vi "Dashboard Main.vi"() -> ()   [LabVIEW 2020]
uses:
  Auto Selector.ctl
  <vilib>/Utility/miscctls.llb/LVRowAndColumnTypeDef.ctl
  <vilib>/event_ctls.llb/eventvkey.ctl
  <vilib>/Rock Robotics/Network Tables/NT Read Numeric Array.vi
  <vilib>/Rock Robotics/Network Tables/NT Read Boolean.vi
  <vilib>/Rock Robotics/WPI/Dashboard/WPI_DashboardLogging Global.vi
panel:
  in  "Camera Settings Right":T1={"Frame Rate"=30, "Compression"=30, "Size"=1, "DB Camera Config"=FALSE} {"Frame Rate" scale=1.0..30.0; "Compression" scale=100.0..-1.0; "Size" items=["640x480", "320x240", "160x120"]}
  in  "Camera Name Right":string(combo)="No Camera Selection"
  in  "Camera Settings":T1={"Frame Rate"=30, "Compression"=30, "Size"=1, "DB Camera Config"=FALSE} {"Frame Rate" scale=1.0..30.0; "Compression" scale=100.0..-1.0; "Size" items=["640x480", "320x240", "160x120"]}
  in  "TCP":refnum<k5>
  in  "Rec Mode":enum32{"Stop", "Record", "Playback"}(radio)
  out "Robot IP":string
  out "Image Message":string="Timeout in Camera Communications"
  in  "Dashboard Tab":T2(tab)
  out "Blind Shot":bool
  out "Blind Intake":bool
  in  "Combo Box":string(combo)="Select Autonomous ..."
  in  "WS RPM":dbl=3500.0
  in  "OC RPM":dbl=900.0
  in  "LP RPM":dbl=3900.0
  out "Control Buttons Connected?":bool
  in  "Select Auto":T3="Select Autonomous ..."
  out "NT Connection":bool
  out "MotorChart R":cluster{"Numeric":dbl, "Numeric":dbl}(graph)
  out "MotorChart L":cluster{"Numeric":dbl, "Numeric":dbl}(graph)
  out "MotorSliders R":cluster{"MotorSlide1":dbl, "MotorSlide2":dbl} {"MotorSlide2" scale=-1.0..1.0 scale format="%#_2e"; "MotorSlide1" scale=-1.0..1.0 scale format="%#_2e"}
  out "MotorSliders L":cluster{"MotorSlide1":dbl, "MotorSlide2":dbl} {"MotorSlide2" scale=-1.0..1.0 scale format="%#_2e"; "MotorSlide1" scale=-1.0..1.0 scale format="%#_2e"}
  out "JS1 Z":dbl(slide) scale=-1.0..1.0 scale format="%#_2e"
  out "JS1 Graph":cluster{"X":dbl, "Y":dbl}[](graph)
  out "JS1 Buttons":T4
  out "JS2 Z":dbl(slide) scale=-1.0..1.0 scale format="%#_2e"
  out "JS2 Graph":cluster{"X":dbl, "Y":dbl}[](graph)
  out "JS2 Buttons":T4
  out "Mode":T5(ring)=enum."Auto Disabled"
  out "Right Camera Perf":cluster{"Bandwidth (Mbps)":dbl, "FPS":dbl}
  out "Camera Perf":string
  out "RPM":dbl
  out "BB1":bool
  out "BB 2":bool
  out "ML":bool
  in  "RPM Control":dbl=3400.0
  out "Invert":bool
  out "Slowmode":bool
  in  "Encoder Dist":dbl=80000.0
  out "Missed Mag":bool
  out "RPM Good":bool
  in  "Limelight On":bool
  out "Camera Image Right":T6(plugin-control)
  in  "DB/String 9":string
  in  "DB/String 8":string
  in  "DB/String 7":string
  in  "DB/String 6":string
  in  "DB/String 5":string
  in  "DB/String 4":string
  in  "DB/String 3":string
  in  "DB/String 2":string
  in  "DB/String 1":string
  in  "DB/String 0":string
  in  "DB/Slider 0":dbl(slide) scale=0.0..5.0
  in  "DB/Slider 1":dbl(slide) scale=0.0..5.0
  in  "DB/Slider 2":dbl(slide) scale=0.0..5.0
  in  "DB/Slider 3":dbl(slide) scale=0.0..5.0
  out "DB/LED 3":bool
  out "DB/LED 2":bool
  out "DB/LED 1":bool
  out "DB/LED 0":bool
  in  "DB/Button 3":bool
  in  "DB/Button 2":bool
  in  "DB/Button 1":bool
  in  "DB/Button 0":bool caption="New Name"
  in  "Test Slider":dbl(slide) scale=0.0..100.0 scale format="%#_3g"
  in  "On/Off":bool caption="Solenoid"
  in  "Test Name":u16(ring) items=["Select the test to run..."]
  in  "Test Tree":string(tree)
  in  "Motor":cluster{"Value":dbl, "Enable":bool} {"Value" scale=-1.0..1.0 scale format="%#_3g"}
  out "Progress":T7 {"Test Progress" scale=0.0..100.0}
  in  "Rev/Fwd":cluster{"Forward":bool, "Reverse":bool}
  in  "Test Ring":u16(ring) items=["Monochrome", "Color"]
  out "Cmd Status":string
  in  "Execute Command":bool
  in  "Command Params":string[][](table)
  in  "Command Selection":i32(listbox)
  in  "CheckList":i32(listbox)
  out "Tree":string(tree)
  out "Camera Image":T6(plugin-control)
  out "Background":bool
  in  "Camera Name":string(combo)="No Camera Selection"
  # "HW"
  # "HW"
  # "Joysticks"
  # "Drive Motors"
  # "Front"
  # "Right"
  # "Left"
  # "Back"
  # "This tab is a great place for autonomous settings and robot-specific values.\nPlace controls and indicators inside this tab and match name to\nDashboard Variables on robot. You can also delete this comment."
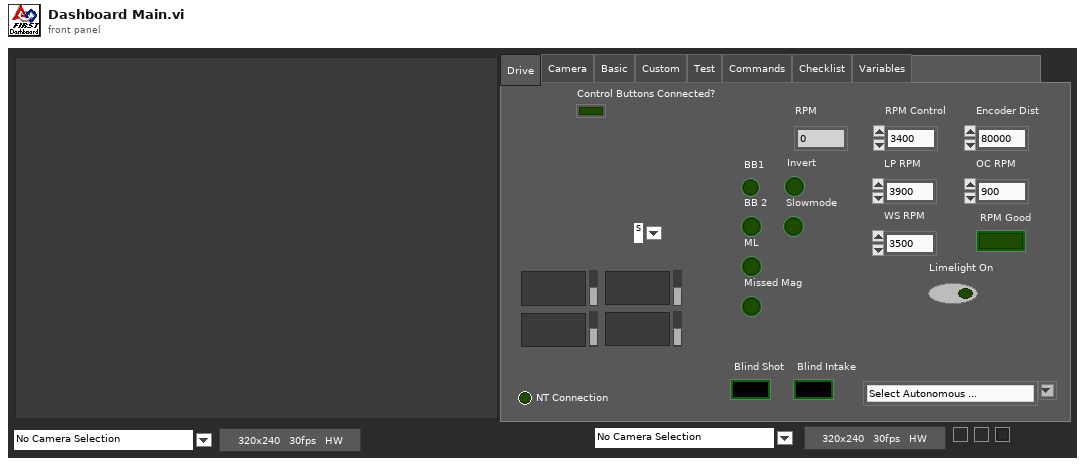
[diagram p1: front panel]
types:
  T1 = cluster{"Frame Rate":i32, "Compression":i32, "Size":u16, "DB Camera Config":bool}
  T2 = enum32{"Drive", "Camera", "Basic", "Custom", "Test", "Commands", "Checklist", "Variables"}
  T3 = typedef "Auto Selector.ctl" = string
  T4 = cluster{bool, bool, bool, bool, bool, bool, bool, bool, bool, bool, bool, bool}
  T5 = enum8{"Tele-Op Disabled", "Tele-Op Enabled", "Auto Disabled", "Auto Enabled", "Test Disabled", "Test Enabled", "Disconnected", "No Code", "E-Stop"}
  T6 = typedef "IMAQ Image.ctl" = refnum<image>
  T7 = cluster{"Test Progress":u8, "Test Progress Text":string}
  T8 = cluster{"Save Path":path, "Interval (s)":dbl, "Keep":i32}
  T9 = typedef "Image Type" = u32
  T10 = cluster{"IDs":cluster{"RPC field ID":u16, "Unique ID":u16}, "String":string}
  T11 = cluster{"Global Rectangle":i32[], "Contours":cluster{"Contour Type":u32, "ROI Type":u32, "Points":i32[]}[]}
  T12 = cluster{"Camera Name":string, string, "Saved DB Images Info":cluster{"Save Path":path, "Interval (s)":dbl, "Keep":i32}}
  T13 = cluster{"Camera Image":refnum<vi>, "Dashboard Tab":refnum<vi>, "Background":refnum<vi>, "Rec Mode":refnum<vi>, "Test Slider":refnum<vi>, "On/Off ":refnum<vi>, "Test Ring":refnum<vi>, "Rev/Fwd":refnum<vi>, "Test Name":refnum<vi>, "Motor":refnum<vi>, "Progress":refnum<vi>, "CheckList":refnum<vi>, "Tree":refnum<vi>, "Test Tree":refnum<vi>, "Command Params":refnum<vi>, "Command Selection":refnum<vi>, "Execute Command":refnum<vi>, "Cmd Status":refnum<vi>, "Camera Settings":refnum<vi>, "Camera Name":refnum<vi>, "Camera Perf":refnum<vi>, "Camera Settings Right":refnum<vi>, "Camera Name Right":refnum<vi>, "Camera Image Right":refnum<vi>}
  T14 = cluster{"Error Strings":string, "Disable Counts":cluster{u16, u16}, "Rail Faults":cluster{u16, u16, u16}, "Robot IP":string, "DB Mode":u8, "Event Info":cluster{"Name":string, "Type":u8, "Number":u16, "Replay":u8}}
  T15 = cluster{"Storage":cluster{"Disk Free":u64, "RAM Block":u32, "RAM free":u32}, "CPU Utilization":cluster{"CPU % ISR":sgl, "CPU % Time Crit":sgl, "CPU % Timed Str":sgl, "CPU % High":sgl, "CPU % Above":sgl, "CPU % Normal":sgl, "CPU % Low":sgl}, "CAN":cluster{"% Bus Utilization":sgl, "Bus Off Cnt":u32, "TX_FIFO Full Cnt":u32, "Receive Error Cnt":u8, "Transmit Error Cnt":u8}, "HID":cluster{"HID Outputs":u32, "Rumble Low":u16, "Rumble High":u16}[]}
  T16 = cluster{"Status bits":cluster{"Test Mode":bool, "Autonomous":bool, "Enabled":bool, "Code Start":bool, "Brownout":bool, "Reserved 2":bool, "Reserved 3":bool, "E-Stop":bool}, "Code Trace":cluster{"Disabled":bool, "TeleOp":bool, "Auto":bool, "Test":bool}, "Controller Type":enum16{"unknown", "cRIO", "roboRio"}, "Code?":enum16{"unknown", "noCode", "code"}, "Battery V":dbl}
  T17 = cluster{"Control Bits":cluster{"TestMode":bool, "Autonomous":bool, "Enabled":bool, "FMS Present":bool, bool, bool, bool, "E-Stop":bool}, "Team Station ":u8, "Countdown":sgl, "Joystick Values":cluster{"Axes":dbl[], "Buttons":bool[], "POVs":i16[]}[]}
  T18 = cluster{"Axes":dbl[], "Buttons":bool[], "POVs":i16[]}[]
  T19 = cluster{"Axes":dbl[], "Buttons":bool[], "POVs":i16[]}
  T20 = cluster{"Buttons[0]":bool, "Buttons[1]":bool, "Buttons[2]":bool, "Buttons[3]":bool, "Buttons[4]":bool, "Buttons[5]":bool, "Buttons[6]":bool, "Buttons[7]":bool, "Buttons[8]":bool, "Buttons[9]":bool, "Buttons[10]":bool, "Buttons[11]":bool}
  T21 = cluster{"Camera Name Right":string, string, "Saved DB Images Info":cluster{"Save Path":path, "Interval (s)":dbl, "Keep":i32}}
  T22 = cluster{"Operation":enum16{"Update", "Clear"}, "Color Box":u32}[]
  T23 = typedef "eventvkey.ctl" = enum16{"ASCII", "Enter", "Return", "Shift", "Ctrl", "Alt", "Cmd", "Opt", "Caps", "NumLock", "Clear", "Break", "Up", "Down", "Left", "Right", "Insert", "Delete", "Home", "End", "PageUp", "PageDown", "Escape", "Help", "Pause", "ScrollLock", "F1", "F2", "F3", "F4", "F5", "F6", "F7", "F8", "F9", "F10", "F11", "F12", "F13", "F14", "F15", "F16", "F17", "F18", "F19", "F20", "F21", "F22", "F23", "F24", "Play", "VolumeUp", "VolumeDown", "Mute", "Two Byte Char"}
  T24 = cluster{"Image Size":bool, "Image Type":bool, "Pixel Value":bool, "ROI Information":bool, "Zoom Factor":bool}
  T25 = cluster{"Operation":enum16{"Update", "Clear"}, "Color Box":u32}
  T26 = typedef "LVRowAndColumnTypeDef.ctl" = cluster{"Row":i32, "Column":i32}
  T27 = cluster{"Shift":bool, "Ctrl":bool, "Alt":bool, "Cmd":bool, "Opt":bool}
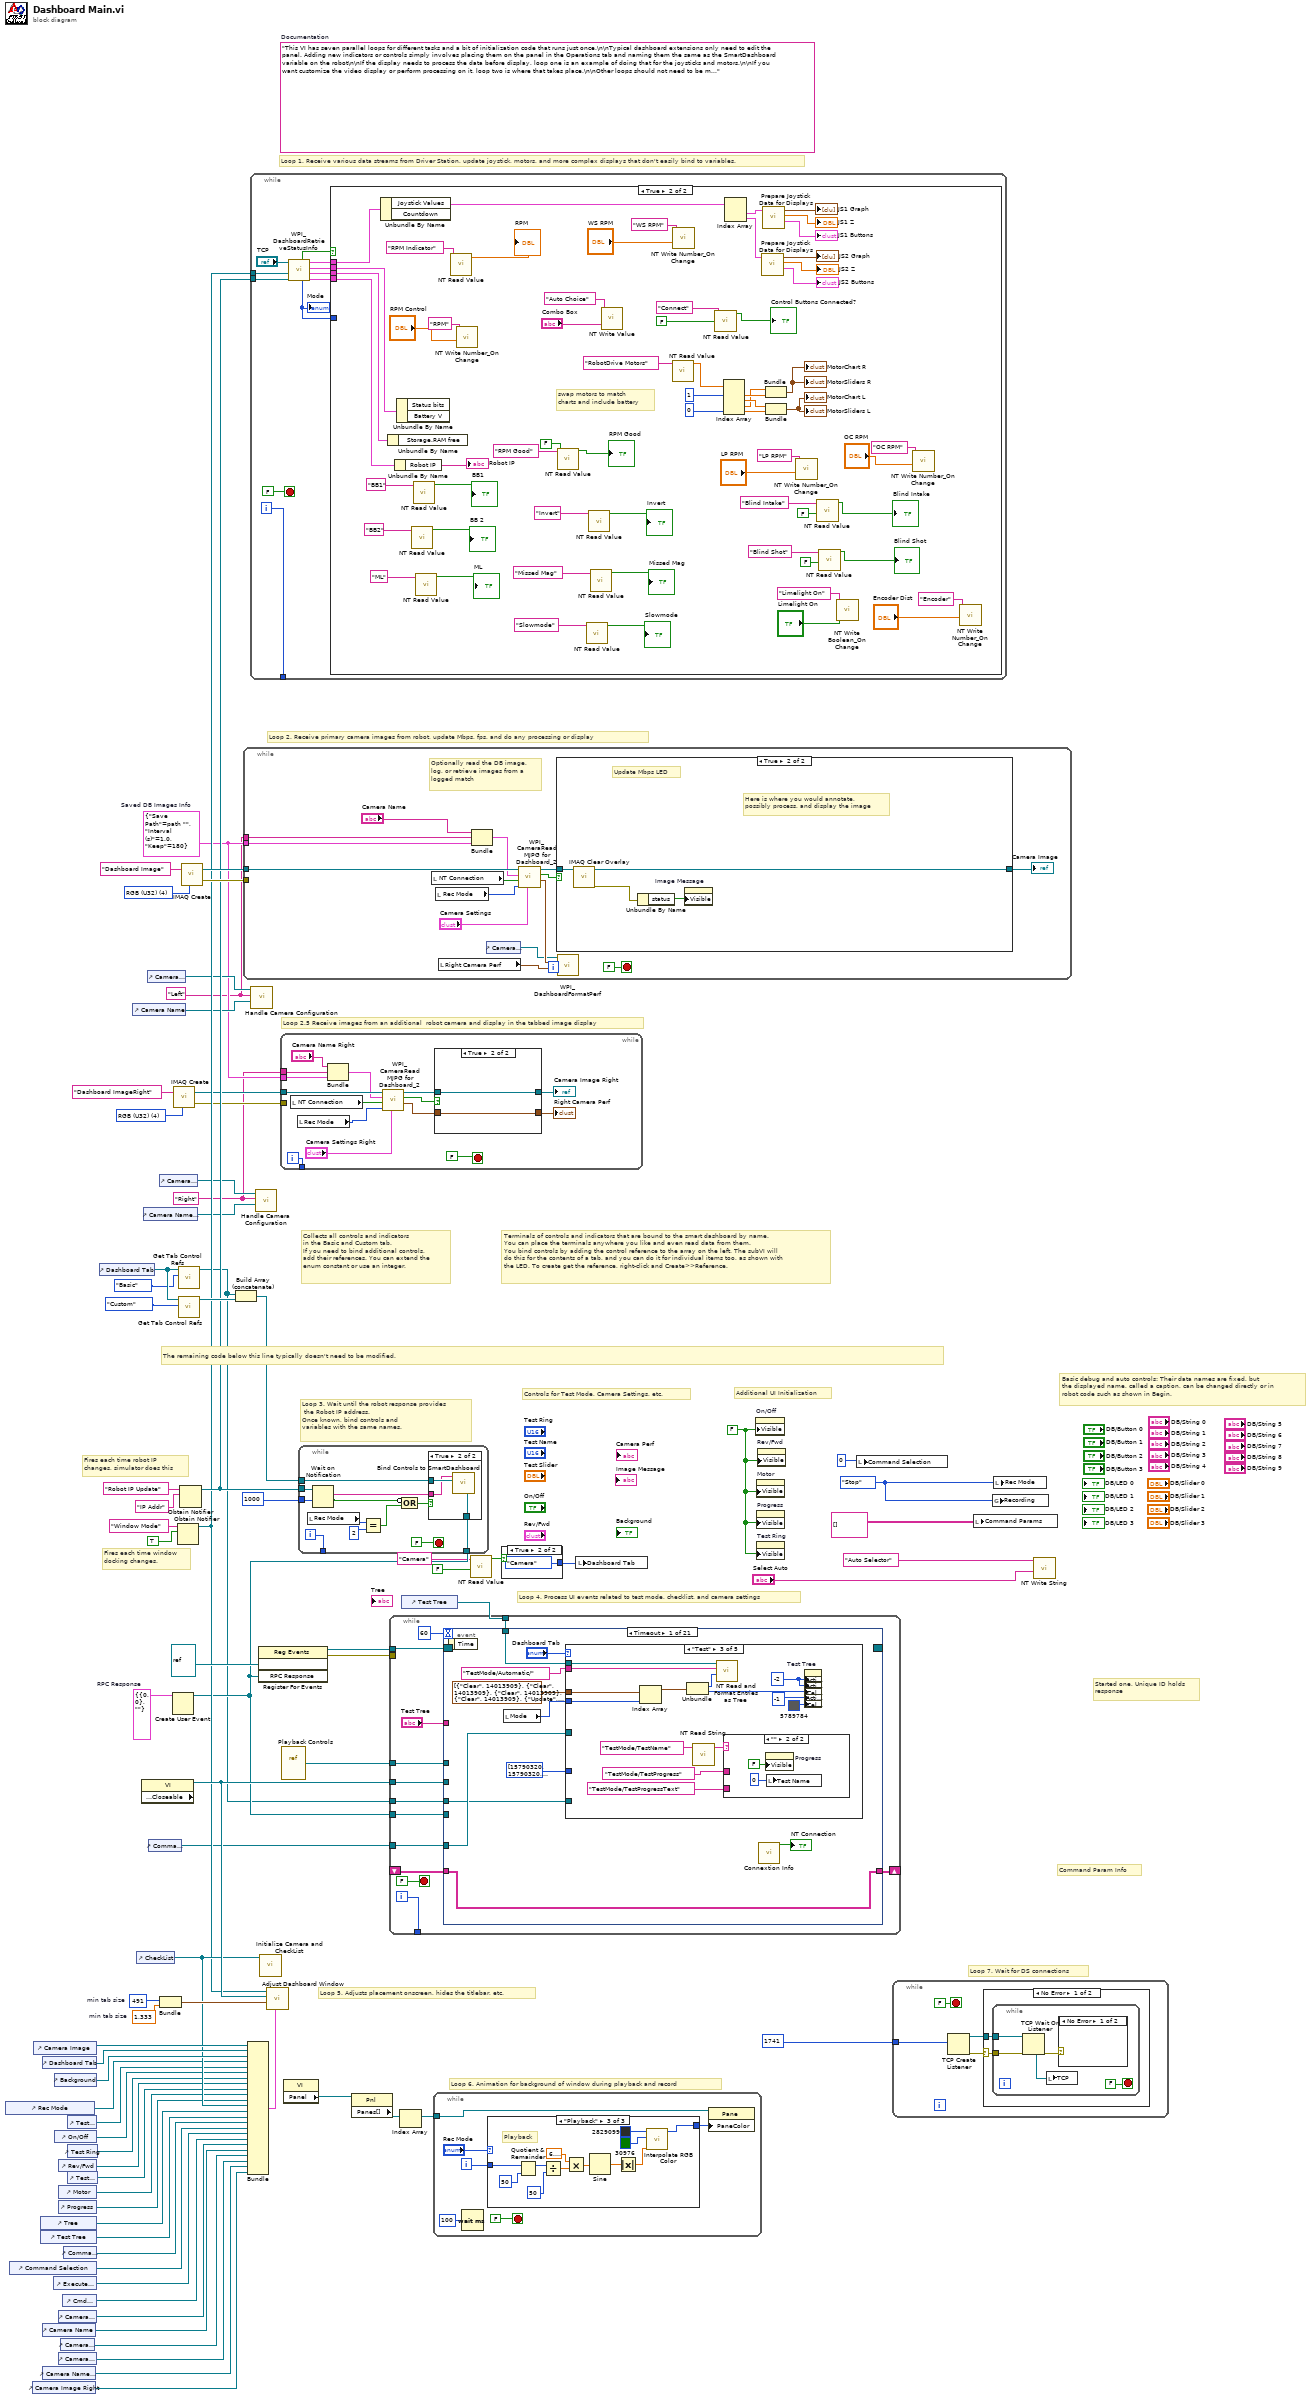
[diagram p0: block diagram]
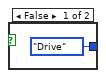
[diagram p2: hidden frame]
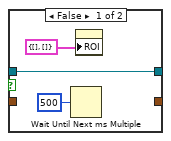
[diagram p3: hidden frame]
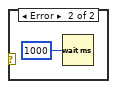
[diagram p4: hidden frame]
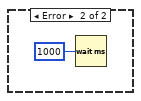
[diagram p5: hidden frame]
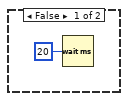
[diagram p6: hidden frame]
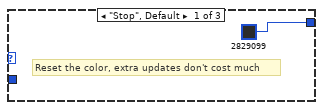
[diagram p7: hidden frame]
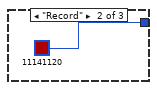
[diagram p8: hidden frame]
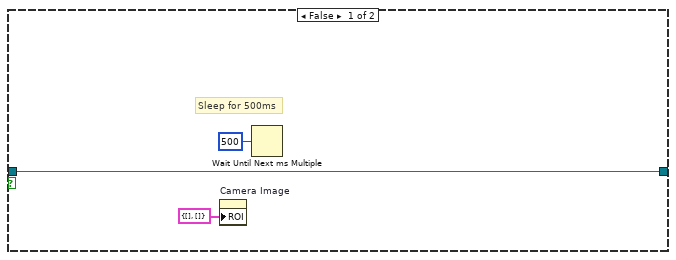
[diagram p10: hidden frame]
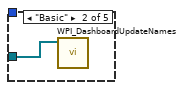
[diagram p12: hidden frame]
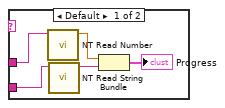
[diagram p13: hidden frame]
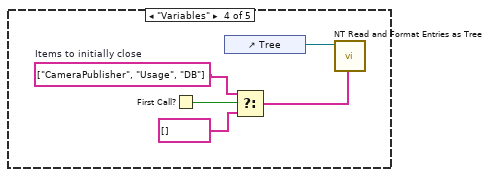
[diagram p14: hidden frame]
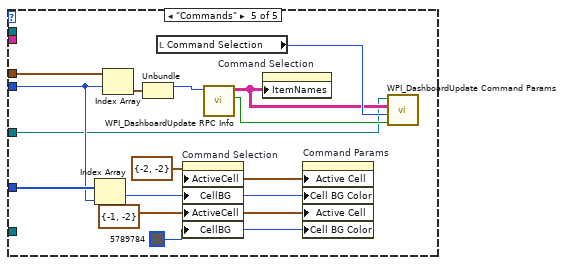
[diagram p15: hidden frame]
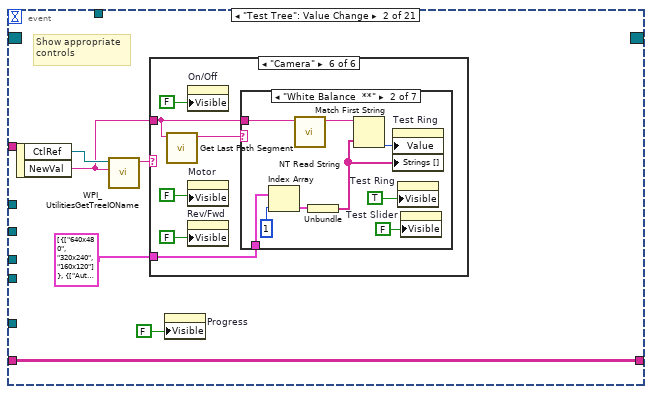
[diagram p16: hidden frame]
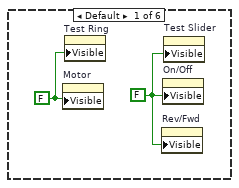
[diagram p17: hidden frame]
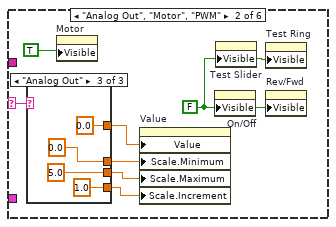
[diagram p18: hidden frame]
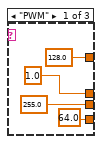
[diagram p19: hidden frame]
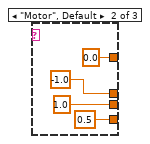
[diagram p20: hidden frame]
diagram:
  w7 = T8 {"Save Path"=path "", "Interval (s)"=1.0, "Keep"=180}  # Saved DB Images Info
  w6 = "Right"
  w5 = "Left"
  w17 = T9 4 items=["Grayscale (U8)", "Grayscale (I16)", "Grayscale (SGL)", "Complex (CSG)", "RGB (U32)", "HSL (U32)", "RGB (U64)"] ("Image Type")
  w32 = T10 {"IDs"={"RPC field ID"=0, "Unique ID"=0}, "String"=""}  # RPC Response
  w55 = 491  # min tab size
  w54 = 1.333  # min tab size
  w62 = enum32{"Stop", "Record", "Playback"}."Stop" ("Rec Mode")
  w39 = FALSE ("Visible")
  (unwired) "This VI has seven parallel loops for different tasks and a bit of initialization code that runs just once.\n\nTypical dashboard extensions only need to edit the panel. Adding new indicators or controls simply involves placing them on the panel in the Operations tab and naming them the same as the SmartDashboard variable on the robot\n\nIf the display needs to process the data before display, loop one is an example of doing that for the joysticks and motors.\n\nIf you want customize the video display or perform processing on it, loop two is where that takes place.\n\nOther loops should not need to be modified. They are pretty standard, and document the task they perform."  # Documentation
  w79 = T9 4 items=["Grayscale (U8)", "Grayscale (I16)", "Grayscale (SGL)", "Complex (CSG)", "RGB (U32)", "HSL (U32)", "RGB (U64)"] ("Image Type")
  # "Loop 2.5 Receive images from an additional  robot camera and display in the tabbed image display"
  # "Command Param Info"
  # "Started one, Unique ID holds\nresponse"
  # "Loop 7. Wait for DS connections"
  # "Basic debug and auto controls: Their data names are fixed, but\nthe displayed name, called a caption, can be changed directly or in\nrobot code such as shown in Begin."
  # "Controls for Test Mode, Camera Settings, etc."
  # "Additional UI Initialization"
  # "Loop 6. Animation for background of window during playback and record"
  # "Fires each time robot IP\nchanges, simulator does this"
  # "Fires each time window\ndocking changes."
  # "Collects all controls and indicators\nin the Basic and Custom tab.\nIf you need to bind additional controls,\nadd their references. You can extend the\nenum constant or use an integer."
  # "The remaining code below this line typically doesn't need to be modified."
  # "Loop 4. Process UI events related to test mode, checklist, and camera settings"
  # "Terminals of controls and indicators that are bound to the smart dashboard by name.\nYou can place the terminals anywhere you like and even read data from them.\nYou bind controls by adding the control reference to the array on the left. The subVI will\ndo this for the contents of a tab, and you can do it for individual items too, as shown with\nthe LED. To create get the reference, right-click and Create>>Reference."
  # "Loop 3. Wait until the robot response provides\n the Robot IP address.\nOnce known, bind controls and\nvariables with the same names."
  # "Loop 5. Adjusts placement onscreen, hides the titlebar, etc."
  # "Loop 1. Receive various data streams from Driver Station, update joystick, motors, and more complex displays that don't easily bind to variables."
  # "Loop 2. Receive primary camera images from robot, update Mbps, fps, and do any processing or display"
  n1 = control-ref of="Rec Mode"() -> (w45:refnum<vi>)
  n2 = control-ref of="Command Selection"() -> (w31:refnum<vi>)
  n3 = control-ref of="Camera Image Right"() -> (w10:refnum<vi>)
  n4 = control-ref of="Camera Image"() -> (w57:refnum<vi>)
  n5 = control-ref of="Tree"() -> (w49:refnum<vi>)
  n6 = control-ref of="Test Tree"() -> (w48:refnum<vi>)
  n7 = control-ref of="Dashboard Tab"() -> (w56:refnum<vi>)
  n8 = control-ref of="Camera Name"() -> (w4:refnum<vi>)
  n9 = control-ref of="Camera Name Right"() -> (w11:refnum<vi>)
  n10 = control-ref of="Execute Command"() -> (w33:refnum<vi>)
  n11 = control-ref of="Background"() -> (w52:refnum<vi>)
  n12 = control-ref of="On/Off"() -> (w43:refnum<vi>)
  n13 = control-ref of="Progress"() -> (w40:refnum<vi>)
  n14 = control-ref of="Camera Settings"() -> (w23:refnum<vi>)
  n15 = control-ref of="Camera Settings Right"() -> (w12:refnum<vi>)
  n16 = control-ref of="Rev/Fwd"() -> (w41:refnum<vi>)
  n17 = control-ref of="Motor"() -> (w46:refnum<vi>)
  n18 = control-ref of="Camera Perf"() -> (w22:refnum<vi>)
  n19 = control-ref of="Cmd Status"() -> (w27:refnum<vi>)
  n20 = control-ref of="Command Params"() -> (w34:refnum<vi>)
  n21 = control-ref of="Test Slider"() -> (w44:refnum<vi>)
  n22 = control-ref of="Test Ring"() -> (w42:refnum<vi>)
  n23 = control-ref of="Test Name"() -> (w47:refnum<vi>)
  n24 = control-ref of="Dashboard Tab"() -> (w60:refnum<vi>)
  n25 = control-ref of="Camera Name"() -> (w24:refnum<vi>)
  n26 = control-ref of="CheckList"() -> (w50:refnum<vi>)
  n27 = property class="VI" props=["Front Panel.Closeable"]() -> (reference out=w61:refnum<vi>)  [unwired: 2 in, 2 out]
  n28 = control-ref of="Camera Name Right"() -> (w13:refnum<vi>)
  n29 = control-ref of="Camera Settings"() -> (w25:refnum<vi>)
  n30 = control-ref of="Command Params"() -> (w26:refnum<vi>)
  n31 = control-ref of="Camera Settings Right"() -> (w14:refnum<vi>)
  n32 = Bundle("min tab size"=w55, "min tab size"=w54) -> (w53:cluster{"min tab size":i32, "min tab size":dbl})  [unwired: 1 in]
  n33 = Create User Event(user event datatype=w32) -> (user event=w28:refnum<user-event>)  [unwired: 1 in, 1 out]
  n34 = call "IMAQ Create"("Image Name"="Dashboard ImageRight", "Image Type"=w17) -> ("New Image"=w16:T6, "error out"=w15:errorcluster)  [unwired: 2 in, 1 out]
  n35 = Obtain Notifier(name (unnamed)="Window Mode", notification data type=TRUE) -> (notifier out=w37:refnum<notifier>)  [unwired: 2 in, 2 out]
  n36 = call <vilib>:"Get Tab Control Refs.vi"("Page Index"=T2."Basic" ("Dashboard Tab"), "TabControl in"=w60) -> ("ControlsOnPage"=w21:refnum<vi>[])  [unwired: 9 in]
  n37 = call <vilib>:"Get Tab Control Refs.vi"("Page Index"=T2."Custom" ("Dashboard Tab"), "TabControl in"=w60) -> ("ControlsOnPage"=w59:refnum<vi>[])  [unwired: 9 in]
  n38 = Obtain Notifier(name (unnamed)="Robot IP Update", notification data type="IP Addr" ("name (unnamed)")) -> (notifier out=w38:refnum<notifier>)  [unwired: 2 in, 2 out]
  n39 = call "IMAQ Create"("Image Name"="Dashboard Image", "Image Type"=w79) -> ("New Image"=w77:T6, "error out"=w76:errorcluster)  [unwired: 2 in, 1 out]
  n40 = Build Array (concatenate)(w21, w59) -> (w58:refnum<vi>[])
  n41 = while {
    tunnel: w77 -> [w93]
    tunnel: w76 -> [_]
    tunnel: w7 -> [w86]
    tunnel: w5 -> [w84]
    stop <- FALSE stop-if-true
    # "Optionally read the DB image,\nlog, or retrieve images from a\nlogged match"
    n42 = local read "NT Connection"() -> (w87:bool)
    n43 = local read "Rec Mode"() -> (w90:enum32{"Stop", "Record", "Playback"})
    n44 = local read "Right Camera Perf"() -> (w82:cluster{"Bandwidth (Mbps)":dbl, "FPS":dbl})
    n45 = Bundle("Camera Name"="Camera Name", w84, "Saved DB Images Info"=w86) -> (w85:T12)  [unwired: 1 in]
    n46 = control-ref of="Camera Perf"() -> (w81:refnum<vi>)
    n47 = call <vilib>:"WPI_CameraRead MJPG for Dashboard_2.vi"("Camera Settings"="Camera Settings", "Rec Mode"=w90, "NT Connection"=w87, "Capture Info"=w85, "Image in"=w93) -> ("perf info"=w83:cluster{"Bandwidth (Mbps)":dbl, "fps":dbl}, "Active"=w91:bool, "Image\\ out"=w92:T6)  [unwired: 4 in]
    n48 = case shown="True" w91 {
      tunnel: w92 -> [w96 w99]
      tunnel: [w96 w98] -> w88
      frame False {
        # "Sleep for 500ms"
        n49 = property on="Camera Image" class="ImageControl"("ROI"=T11 {"Global Rectangle"=[], "Contours"=[]}) -> ()  [unwired: 2 in, 2 out]
        n50 = Wait Until Next ms Multiple(millisecond multiple=u32 500) -> ()  [unwired: 1 out]
      }
      frame True {
        # "Here is where you would annotate,\npossibly process, and display the image"
        # "Update Mbps LED"
        n51 = call "IMAQ Clear Overlay"("Image"=w99) -> ("error out"=w100:errorcluster, "Image Out"=w98:T6)  [unwired: 2 in, 7 out]
        n52 = Unbundle By Name(w100) -> ("status"=w101:bool)
        n53 = property on="Image Message" class="Str"("Visible"=w101) -> ()  [unwired: 2 in, 2 out]
      }
    }
    "Camera Image" <- w88
    n54 = call <vilib>:"WPI_DashboardFormatPerf.vi"("Right Camera Perf"=w82, "Performance"=w83, "String in"=w81) -> ()  [unwired: 9 in]
  }
  n55 = Bundle("Camera Image"=w57, "Dashboard Tab"=w56, "Background"=w52, "Rec Mode"=w45, "Test Slider"=w44, "On/Off"=w43, "Test Ring"=w42, "Rev/Fwd"=w41, "Test Name"=w47, "Motor"=w46, "Progress"=w40, "CheckList"=w50, "Tree"=w49, "Test Tree"=w48, "Command Params"=w34, "Command Selection"=w31, "Execute Command"=w33, "Cmd Status"=w27, "Camera Settings"=w23, "Camera Name"=w4, "Camera Perf"=w22, "Camera Settings Right"=w12, "Camera Name Right"=w11, "Camera Image Right"=w10) -> (w51:T13)  [unwired: 1 in]
  n56 = while {
    tunnel: [w111] -> _
    tunnel: w38 -> [w105]
    tunnel: w37 -> [w102]
    i -> [w111]
    stop <- FALSE stop-if-true
    n57 = call <vilib>:"WPI_DashboardRetrieveStatusInfo.vi"("Binding Refnum"=w105, "Window Mode Notifier"=w102, "TCP Cnx"="TCP") -> ("Power and Errors"=w106:T14, "Robot Metrics"=w109:T15, "Status Info"=w110:T16, "Control Info"=w107:T17, "Robot Mode"=w104:T5, "Process?"=w108:bool)  [unwired: 3 in]
    "Mode" <- w104
    n58 = case shown="True" w108 {
      tunnel: w110 -> [_ w177]
      tunnel: w109 -> [_ w176]
      tunnel: w107 -> [_ w175]
      tunnel: w106 -> [_ w174]
      tunnel: w104 -> [_ _]
      frame False {
        n59 = Wait (ms)(milliseconds to wait=u32 20) -> ()  [unwired: 1 out]
      }
      frame True {
        # "swap motors to match\ncharts and include battery"
        n60 = Unbundle By Name(w175) -> ("Joystick Values"=w165:T18)  [unwired: 1 out]
        n61 = Unbundle By Name(w176) -> ()  [unwired: 1 out]
        n62 = Unbundle By Name(w174) -> ("Robot IP"=→"Robot IP":string)
        n63 = Unbundle By Name(w177) -> ()  [unwired: 2 out]
        n64 = call-poly <vilib>:"NT Read Value.vi"("Name"="BB2") -> ("Boolean"=→"BB 2":bool)  [unwired: 9 in, 1 out]
        n65 = call-poly <vilib>:"NT Read Value.vi"("Name"="BB1") -> ("Boolean"=→"BB1":bool)  [unwired: 9 in, 1 out]
        n66 = call-poly <vilib>:"NT Read Value.vi"("Name"="ML") -> ("Boolean"=→"ML":bool)  [unwired: 9 in, 1 out]
        n67 = call-poly <vilib>:"NT Read Value.vi"("Name"="RPM Indicator") -> ("Numeric"=→"RPM":dbl)  [unwired: 9 in, 1 out]
        n68 = call "NT Write Number_On Change.vi"("Numeric"="RPM Control", "Name"="RPM") -> ()  [unwired: 9 in, 1 out]
        n69 = call-poly <vilib>:"NT Read Value.vi"("Default Value"=FALSE, "Name"="RPM Good") -> ("Boolean"=→"RPM Good":bool)  [unwired: 8 in, 1 out]
        n70 = call-poly <vilib>:"NT Read Value.vi"("Name"="Slowmode") -> ("Boolean"=→"Slowmode":bool)  [unwired: 9 in, 1 out]
        n71 = call-poly <vilib>:"NT Read Value.vi"("Name"="Invert") -> ("Boolean"=→"Invert":bool)  [unwired: 9 in, 1 out]
        n72 = call-poly <vilib>:"NT Read Value.vi"("Name"="Missed Mag") -> ("Boolean"=→"Missed Mag":bool)  [unwired: 9 in, 1 out]
        n73 = call-poly <vilib>:"NT Write Value.vi"("String"="Combo Box", "Name"="Auto Choice") -> ()  [unwired: 9 in, 1 out]
        n74 = call-poly <vilib>:"NT Read Value.vi"("Name"="RobotDrive Motors") -> ("Numeric Array"=w155:dbl[])  [unwired: 9 in, 1 out]
        n75 = call "NT Write Number_On Change.vi"("Numeric"="WS RPM", "Name"="WS RPM") -> ()  [unwired: 9 in, 1 out]
        n76 = call-poly <vilib>:"NT Read Value.vi"("Default Value"=FALSE, "Name"="Connect") -> ("Boolean"=→"Control Buttons Connected?":bool)  [unwired: 8 in, 1 out]
        n77 = Index Array(array=w155, index #1=1, index #4=0) -> (element #1=w169:dbl, element #2=w170:dbl, element #3=w168:dbl, element #4=w173:dbl)  [unwired: 2 in]
        n78 = Index Array(array=w165) -> (element #1=w164:T19, element #2=w160:T19)  [unwired: 2 in]
        n79 = call "Prepare Joystick Data for Displays.vi"("Joystick Values"=w160) -> ("Buttons"=→"JS2 Buttons":T20, "Z Axis"=→"JS2 Z":dbl, "Cartesian Data"=→"JS2 Graph":cluster{"X axis":dbl, "X axis":dbl}[])  [unwired: 8 in]
        n80 = call "Prepare Joystick Data for Displays.vi"("Joystick Values"=w164) -> ("Buttons"=→"JS1 Buttons":T20, "Z Axis"=→"JS1 Z":dbl, "Cartesian Data"=→"JS1 Graph":cluster{"X axis":dbl, "X axis":dbl}[])  [unwired: 8 in]
        n81 = Bundle("Numeric"=w168, "Numeric"=w169) -> (→"MotorChart R" →"MotorSliders R":cluster{"Numeric":dbl, "Numeric":dbl})  [unwired: 1 in]
        n82 = Bundle("Numeric"=w170, "Numeric"=w173) -> (→"MotorChart L" →"MotorSliders L":cluster{"Numeric":dbl, "Numeric":dbl})  [unwired: 1 in]
        n83 = call "NT Write Number_On Change.vi"("Numeric"="LP RPM", "Name"="LP RPM") -> ()  [unwired: 9 in, 1 out]
        n84 = call-poly <vilib>:"NT Read Value.vi"("Default Value"=FALSE, "Name"="Blind Intake") -> ("Boolean"=→"Blind Intake":bool)  [unwired: 8 in, 1 out]
        n85 = call-poly <vilib>:"NT Read Value.vi"("Default Value"=FALSE, "Name"="Blind Shot") -> ("Boolean"=→"Blind Shot":bool)  [unwired: 8 in, 1 out]
        n86 = call "NT Write Boolean_On Change.vi"("Boolean"="Limelight On", "Name"="Limelight On") -> ()  [unwired: 9 in, 1 out]
        n87 = call "NT Write Number_On Change.vi"("Numeric"="OC RPM", "Name"="OC RPM") -> ()  [unwired: 9 in, 1 out]
        n88 = call "NT Write Number_On Change.vi"("Numeric"="Encoder Dist", "Name"="Encoder") -> ()  [unwired: 9 in, 1 out]
      }
    }
  }
  n89 = call "Handle Camera Configuration.vi"("CameraNameRef"=w24, "Display Name"=w5, "ClusterRef"=w25) -> ()  [unwired: 9 in]
  n90 = call "Handle Camera Configuration.vi"("CameraNameRef"=w13, "Display Name"=w6, "ClusterRef"=w14) -> ()  [unwired: 9 in]
  n91 = register-events(refnum<vi> refnum, w28) -> (reference out=w66:refnum<event-registration>, error out=w65:errorcluster)  [unwired: 2 in]
  n92 = call "Initialize Camera and CheckList.vi"("ListBox in"=w50) -> ()  [unwired: 11 in]
  n93 = call "Adjust Dashboard Window.vi"("Sizing Refnums"=w51, "Size Constraints"=w53, "VI"=w61, "WIn Mode"=w37) -> ()  [unwired: 8 in]
  n94 = while {
    tunnel: w16 -> [w192]
    tunnel: w15 -> [_]
    tunnel: [w187] -> _
    tunnel: w7 -> [w183]
    tunnel: w6 -> [w180]
    i -> [w187]
    stop <- FALSE stop-if-true
    n95 = local read "NT Connection"() -> (w184:bool)
    n96 = local read "Rec Mode"() -> (w191:enum32{"Stop", "Record", "Playback"})
    n97 = Bundle("Camera Name Right"="Camera Name Right", w180, "Saved DB Images Info"=w183) -> (w182:T21)  [unwired: 1 in]
    n98 = call <vilib>:"WPI_CameraRead MJPG for Dashboard_2.vi"("Camera Settings"="Camera Settings Right", "Rec Mode"=w191, "NT Connection"=w184, "Capture Info"=w182, "Image in"=w192) -> ("perf info"=w178:cluster{"Bandwidth (Mbps)":dbl, "fps":dbl}, "Active"=w186:bool, "Image\\ out"=w189:T6)  [unwired: 4 in]
    n99 = case shown="True" w186 {
      tunnel: w189 -> [w194 w197]
      tunnel: [w194 w197] -> w185
      tunnel: [_ w196] -> w179
      tunnel: w178 -> [_ w196]
      frame False {
        n100 = Wait Until Next ms Multiple(millisecond multiple=u32 500) -> ()  [unwired: 1 out]
        n101 = property on="Camera Image Right" class="ImageControl"("ROI"=T11 {"Global Rectangle"=[], "Contours"=[]}) -> ()  [unwired: 2 in, 2 out]
      }
      frame True {
      }
    }
    "Camera Image Right" <- w185
    "Right Camera Perf" <- w179
  }
  n102 = vi-ref "Playback Controls.vi"() -> (w67:refnum<vi>)
  n103 = property class="VI"() -> ("Panel"=w69:refnum<vi>)  [unwired: 2 in, 2 out]
  n104 = while {
    tunnel: w58 -> [w209]
    tunnel: w38 -> [w207]
    tunnel: [w205] -> _
    tunnel: u32 1000 ("milliseconds to wait") -> [w204]
    tunnel: w28 -> [w198]
    i -> [w205]
    stop <- FALSE stop-if-true
    n105 = local read "Rec Mode"() -> (w200:enum32{"Stop", "Record", "Playback"})
    n106 = Wait on Notification(notifier=w207, timeout in ms (-1)=w204) -> (notification=w206:string, timed out?=w202:bool)  [unwired: 2 in, 2 out]
    n107 = Equal?(x=w200, y=u16 2 ("Rec Mode")) -> (x = y?=w201:bool)
    n108 = Compound Arithmetic op=OR(invert w202, w201) -> (w203:bool)
    n109 = case shown="True" w203 {
      tunnel: w209 -> [_ w212]
      tunnel: w206 -> [_ w211]
      tunnel: w198 -> [_ w210]
      frame False {
      }
      frame True {
        n110 = call <vilib>:"Bind Controls to SmartDashboard.vi"("RPC ref"=w210, "Bound Control Refs"=w212, "Server IP Address"=w211) -> ()  [unwired: 9 in]
      }
    }
  }
  n111 = property class="Pnl"(reference=w69) -> ("Panes[]"=w70:refnum<vi>[])  [unwired: 1 in, 2 out]
  n112 = Index Array(array=w70) -> (element=w68:refnum<vi>)  [unwired: 1 in]
  n113 = control-ref of="Test Tree"() -> (w71:refnum<vi>)
  n114 = while {
    tunnel: [w222] -> _
    tunnel: w71 -> [w221]
    tunnel: w67 -> [w220]
    tunnel: w66 -> [w219]
    tunnel: w65 -> [_]
    tunnel: w61 -> [w218]
    tunnel: w28 -> [w217]
    tunnel: w26 -> [w216]
    shift-right: [w215] -> _
    shift-left: _ -> [w214]
    tunnel: w21 -> [w213]
    i -> [w222]
    stop <- FALSE stop-if-true
    n115 = event shown="[0] Timeout" {
      selector: w219 -> [_ _ _ _ _ _ _ _ _ _ _ _ _ _ _ _ _ _ _ _ _]
      dyn-events: [_ _ _ _ _ _ _ _ _ _ _ _ _ _ _ _ w482 _ _ _ _] -> _
      timeout: u32 60 ("milliseconds to wait") -> [_ _ _ _ _ _ _ _ _ _ _ _ _ _ _ _ _ _ _ _ _]
      tunnel: w221 -> [w234 _ _ _ _ _ _ _ _ _ _ _ _ _ _ _ _ _ _ _ _]
      tunnel: "Test Tree" -> [_ _ _ _ _ _ _ _ _ _ _ w449 w457 w459 w463 w471 _ _ _ _ _]
      tunnel: w220 -> [_ _ _ _ _ _ _ _ _ _ _ _ _ _ _ _ w484 _ w502 _ _]
      tunnel: w218 -> [_ _ _ _ _ _ _ _ _ _ _ _ _ _ _ _ w480 _ _ _ _]
      tunnel: w217 -> [_ _ _ _ _ _ _ _ _ _ _ _ _ _ _ _ w478 _ _ _ _]
      tunnel: w216 -> [w229 _ _ _ _ _ w400 _ _ _ _ _ _ _ _ _ _ _ _ _ _]
      tunnel: [w228 w277 w379 w384 w393 w397 w398 w407 w417 w424 w436 w448 w455 w458 w462 w470 w477 w497 w499 w503 w516] -> w215
      tunnel: w214 -> [w228 w277 w379 w384 w393 w397 w398 _ _ w424 w436 w448 w455 w458 w462 w470 w477 w497 w499 w503 w516]
      tunnel: w213 -> [w226 _ _ _ _ _ _ _ _ _ _ _ _ _ _ _ _ _ _ _ _]
      event Timeout {
        n116 = event-data() -> ()  [unwired: 1 in, 1 out]
        n117 = local read "Mode"() -> (w231:T5)
        n118 = case shown="\"Test\"" "Dashboard Tab" {
          tunnel: w234 -> [_ _ w250 _ _]
          tunnel: "TestMode/Automatic/" ("Name Pattern") -> [_ _ w249 _ _]
          tunnel: T22 [{"Operation"=enum."Clear", "Color Box"=14013909}, {"Operation"=enum."Clear", "Color Box"=14013909}, {"Operation"=enum."Clear", "Color Box"=14013909}, {"Operation"=enum."Clear", "Color Box"=14013909}, {"Operation"=enum."Update", "Color Box"=14013909}, {"Operation"=enum."Update", "Color Box"=16777215}, {"Operation"=enum."Clear", "Color Box"=14013909}, {"Operation"=enum."Clear", "Color Box"=14013909}, {"Operation"=enum."Clear", "Color Box"=14013909}] -> [_ _ w242 _ w270]
          tunnel: w231 -> [_ _ w241 _ w269]
          tunnel: u32[] [15790320, 15790320, 15790320, 15790320, 16777215, 16777215, 15790320, 15790320, 15790320] -> [_ _ _ _ w275]
          tunnel: w229 -> [_ _ _ _ w263]
          tunnel: w226 -> [_ w236 _ _ _]
          frame "Custom", Default {
          }
          frame "Basic" {
            n119 = call <vilib>:"WPI_DashboardUpdateNames.vi"("Controls on Tab"=w236) -> ()  [unwired: 11 in]
          }
          frame "Test" {
            w248 = -2 ("Active Item:Row Number")
            n120 = Index Array(array=w242, index=w241) -> (element=w243:T25)
            n121 = Unbundle(w243) -> ("Operation"=w244:enum16{"Update", "Clear"}, "Color Box"=w245:u32)
            n122 = call <vilib>:"NT Read String.vi"("Name"="TestMode/TestName") -> ("String"=w239:string)  [unwired: 9 in, 1 out]
            n123 = call <vilib>:"NT Read and Format Entries as Tree.vi"("Operation"=w244, "Name Pattern"=w249, "Tree Refnum"=w250) -> ()  [unwired: 7 in, 2 out]
            n124 = case shown="\"\"" w239 {
              tunnel: "TestMode/TestProgress" ("Name") -> [w252 _]
              tunnel: "TestMode/TestProgressText" ("Name") -> [w251 _]
              frame Default {
                n125 = call <vilib>:"NT Read Number.vi"("Name"=w252) -> ("Numeric"=w253:dbl)  [unwired: 9 in, 1 out]
                n126 = call <vilib>:"NT Read String.vi"("Name"=w251) -> ("String"=w254:string)  [unwired: 9 in, 1 out]
                n127 = Bundle("Numeric"=w253, "String"=w254) -> (→"Progress":cluster{"Numeric":dbl, "String":string})  [unwired: 1 in]
              }
              frame "" {
                n128 = property on="Progress" class="Clust (strict)"("Visible"=FALSE) -> ()  [unwired: 2 in, 2 out]
                n129 = local write "Test Name"(u16 0) -> ()
              }
            }
            n130 = property on="Test Tree" class="Tree (strict)"("Active Item Row Number"=w248, "ActiveColNum"=w248, "CellBG"=w245, "Active Item Row Number"=-1 ("Active Item:Row Number"), "CellBG"=u32 5789784 ("Color Box")) -> ()  [unwired: 2 in, 2 out]
          }
          frame "Variables" {
            w260 = string[] ["CameraPublisher", "Usage", "DB"]  # Items to initially close
            n131 = First Call?() -> (First Call?: T/F=w261:bool)
            n132 = control-ref of="Tree"() -> (w262:refnum<vi>)
            n133 = Select(t=w260, s=w261, f=string[] []) -> (s? t:f=w258:string[])
            n134 = call <vilib>:"NT Read and Format Entries as Tree.vi"("Tags to  Close"=w258, "Tree Refnum"=w262) -> ()  [unwired: 8 in, 2 out]
          }
          frame "Commands" {
            w271 = u32 5789784 ("Color Box")
            w272 = T26 {"Row"=-1, "Column"=-2} ("Active Cell:Active Cell")
            w274 = T26 {"Row"=-2, "Column"=-2} ("Active Cell:Active Cell")
            n135 = Index Array(array=w275, index=w269) -> (element=w273:u32)
            n136 = Index Array(array=w270, index=w269) -> (element=w268:T25)
            n137 = Unbundle(w268) -> ("Operation"=w267:enum16{"Update", "Clear"})  [unwired: 1 out]
            n138 = local read "Command Selection"() -> (w266:i32)
            n139 = property on="Command Selection" class="MCListbox (strict)"("ActiveCell"=w274, "CellBG"=w273, "ActiveCell"=w272, "CellBG"=w271) -> ()  [unwired: 2 in, 2 out]
            n140 = call <vilib>:"WPI_DashboardUpdate RPC Info.vi"("Operation"=w267) -> ("update"=w265:bool, "commands"=w264:string[][])  [unwired: 9 in]
            n141 = property on="Command Selection" class="MCListbox (strict)"("ItemNames"=w264) -> ()  [unwired: 2 in, 2 out]
            n142 = property on="Command Params" class="Tbl (strict)"("Active Cell"=w274, "Cell BG Color"=w273, "Active Cell"=w272, "Cell BG Color"=w271) -> ()  [unwired: 2 in, 2 out]
            n143 = call <vilib>:"WPI_DashboardUpdate Command Params.vi"("Update"=w265, "NewVal"=w266, "Commands"=w264, "Param Tbl"=w263) -> ()  [unwired: 7 in, 1 out]
          }
        }
        n144 = call <vilib>:"Connextion Info.vi"() -> ("Connected"=→"NT Connection":bool)  [unwired: 10 in, 1 out]
      }
      event "Test Tree": Value Change {
        # "Show appropriate\ncontrols"
        n145 = event-data() -> ("CtlRef"=w280:refnum<vi>, "NewVal"=w278:string)  [unwired: 1 in]
        n146 = call <vilib>:"WPI_UtilitiesGetTreeIOName.vi"("NewVal"=w278, "TreeControl in"=w280) -> ("I/O Name"=w281:string)  [unwired: 9 in]
        n147 = case shown="\"Camera\"" w281 {
          selector: w281 -> [_ w288 _ w310 w319 _]
          tunnel: w278 -> [_ _ w307 w309 _ w326]
          tunnel: cluster{string[]}[] [{["640x480", "320x240", "160x120"]}, {["Auto", "Fixed indoor", "Fixed outdoor 1", "Fixed outdoor 2", "Fixed fluorescent 1", "Fixed fluorescent 2", "Hold current"]}, {["Auto", "Flicker-free 50 Hz", "Flicker-free 60 Hz", "Hold current"]}, {["None", "Prioritize frame rate", "Prioritize image quality"]}, {["Monochrome", "Color"]}] -> [_ _ _ _ _ w325]
          frame Default {
            w283 = FALSE ("Visible")
            w282 = FALSE ("Visible")
            n148 = property on="Motor" class="Clust (strict)"("Visible"=w282) -> ()  [unwired: 2 in, 2 out]
            n149 = property on="Test Ring" class="Ring (strict)"("Visible"=w282) -> ()  [unwired: 2 in, 2 out]
            n150 = property on="Rev/Fwd" class="Clust (strict)"("Visible"=w283) -> ()  [unwired: 2 in, 2 out]
            n151 = property on="On/Off" class="Bool (strict)"("Visible"=w283) -> ()  [unwired: 2 in, 2 out]
            n152 = property on="Test Slider" class="Slide (strict)"("Visible"=w283) -> ()  [unwired: 2 in, 2 out]
          }
          frame "Analog Out", "Motor", "PWM" {
            w289 = FALSE ("Visible")
            n153 = case shown="\"Analog Out\"" w288 {
              tunnel: [1.0 ("Value") -1.0 ("Value") 0.0 ("Value")] -> w287
              tunnel: [255.0 ("Value") 1.0 ("Value") 5.0 ("Value")] -> w286
              tunnel: [128.0 ("Value") 0.0 ("Value") 0.0 ("Value")] -> w285
              tunnel: [64.0 ("Value") 0.5 ("Value") 1.0 ("Value")] -> w284
              frame "PWM" {
              }
              frame "Motor", Default {
              }
              frame "Analog Out" {
              }
            }
            n154 = property on="Motor" class="Clust (strict)"("Visible"=TRUE) -> ()  [unwired: 2 in, 2 out]
            n155 = property on="Value" class="Slide (strict)"("Value"=w285, "Scale.Minimum"=w287, "Scale.Maximum"=w286, "Scale.Increment"=w284) -> ()  [unwired: 2 in, 2 out]
            n156 = property on="On/Off" class="Bool (strict)"("Visible"=w289) -> ()  [unwired: 2 in, 2 out]
            n157 = property on="Test Slider" class="Slide (strict)"("Visible"=w289) -> ()  [unwired: 2 in, 2 out]
            n158 = property on="Test Ring" class="Ring (strict)"("Visible"=w289) -> ()  [unwired: 2 in, 2 out]
            n159 = property on="Rev/Fwd" class="Clust (strict)"("Visible"=w289) -> ()  [unwired: 2 in, 2 out]
          }
          frame "Servo" {
            w305 = FALSE ("Visible")
            n160 = call <vilib>:"NT Read Number.vi"("Name"=w307) -> ("Numeric"=w306:dbl)  [unwired: 9 in, 1 out]
            n161 = property on="Test Slider" class="Slide (strict)"("Visible"=TRUE, "Scale.Maximum"=170.0 ("Scale.Range:Maximum")) -> ()  [unwired: 2 in, 2 out]
            n162 = local write "Test Slider"(w306) -> ()
            n163 = property on="Motor" class="Clust (strict)"("Visible"=w305) -> ()  [unwired: 2 in, 2 out]
            n164 = property on="Rev/Fwd" class="Clust (strict)"("Visible"=w305) -> ()  [unwired: 2 in, 2 out]
            n165 = property on="On/Off" class="Bool (strict)"("Visible"=w305) -> ()  [unwired: 2 in, 2 out]
            n166 = property on="Test Ring" class="Ring (strict)"("Visible"=w305) -> ()  [unwired: 2 in, 2 out]
          }
          frame "Relay", "Solenoid" {
            w308 = FALSE ("Visible")
            n167 = property on="Motor" class="Clust (strict)"("Visible"=w308) -> ()  [unwired: 2 in, 2 out]
            n168 = property on="Test Slider" class="Slide (strict)"("Visible"=w308) -> ()  [unwired: 2 in, 2 out]
            n169 = Search and Replace String(input string=w309, search string="/Value  **", replace string="/Direction") -> (result string=w315:string)  [unwired: 5 in, 3 out]
            n170 = property on="Test Ring" class="Ring (strict)"("Visible"=w308) -> ()  [unwired: 2 in, 2 out]
            n171 = call <vilib>:"NT Read String.vi"("Name"=w315) -> ("String"=w313:string)  [unwired: 9 in, 1 out]
            n172 = Equal?(x="Both directions", y=w313) -> (x = y?=w311:bool)
            n173 = Not(x=w311) -> (.not. x?=w312:bool)
            n174 = property on="Rev/Fwd" class="Clust (strict)"("Visible"=w311) -> ()  [unwired: 2 in, 2 out]
            n175 = property on="On/Off" class="Bool (strict)"("Visible"=w312, "Caption.Text"=w310) -> ()  [unwired: 2 in, 2 out]
          }
          frame "Compressor", "Digital Out" {
            w318 = FALSE ("Visible")
            # "Get direction and finish"
            n176 = property on="Motor" class="Clust (strict)"("Visible"=w318) -> ()  [unwired: 2 in, 2 out]
            n177 = property on="Test Slider" class="Slide (strict)"("Visible"=w318) -> ()  [unwired: 2 in, 2 out]
            n178 = property on="Test Ring" class="Ring (strict)"("Visible"=w318) -> ()  [unwired: 2 in, 2 out]
            n179 = property on="On/Off" class="Bool (strict)"("Visible"=TRUE, "Caption.Text"=w319) -> ()  [unwired: 2 in, 2 out]
            n180 = property on="Rev/Fwd" class="Clust (strict)"("Visible"=FALSE) -> ()  [unwired: 2 in, 2 out]
          }
          frame "Camera" {
            n181 = call <vilib>:"Get Last Path Segment.vi"("String in"=w326) -> ("String out"=w327:string)  [unwired: 10 in]
            n182 = property on="On/Off" class="Bool (strict)"("Visible"=FALSE) -> ()  [unwired: 2 in, 2 out]
            n183 = property on="Motor" class="Clust (strict)"("Visible"=FALSE) -> ()  [unwired: 2 in, 2 out]
            n184 = property on="Rev/Fwd" class="Clust (strict)"("Visible"=FALSE) -> ()  [unwired: 2 in, 2 out]
            n185 = case shown="\"White Balance  **\"" w327 {
              tunnel: w326 -> [w333 w342 w351 w360 w369 _ w375]
              tunnel: w325 -> [w331 w339 w348 w357 w366 _ _]
              frame "Size  **" {
                n186 = Index Array(array=w331) -> (element=w330:cluster{string[]})  [unwired: 1 in]
                n187 = call <vilib>:"NT Read String.vi"("Name"=w333) -> ("String"=w332:string)  [unwired: 9 in, 1 out]
                n188 = Unbundle(w330) -> (w328:string[])
                n189 = Match First String(2:w328, 3:w332) -> (0:w329:i32)  [unwired: 1 out]
                n190 = property on="Test Ring" class="Ring (strict)"("Value"=w329, "Strings []"=w328) -> ()  [unwired: 2 in, 2 out]
                n191 = property on="Test Ring" class="Ring (strict)"("Visible"=TRUE) -> ()  [unwired: 2 in, 2 out]
                n192 = property on="Test Slider" class="Slide (strict)"("Visible"=FALSE) -> ()  [unwired: 2 in, 2 out]
              }
              frame "White Balance  **" {
                n193 = Index Array(array=w339, index=1) -> (element=w340:cluster{string[]})
                n194 = call <vilib>:"NT Read String.vi"("Name"=w342) -> ("String"=w341:string)  [unwired: 9 in, 1 out]
                n195 = Unbundle(w340) -> (w337:string[])
                n196 = Match First String(2:w337, 3:w341) -> (0:w336:i32)  [unwired: 1 out]
                n197 = property on="Test Ring" class="Ring (strict)"("Value"=w336, "Strings []"=w337) -> ()  [unwired: 2 in, 2 out]
                n198 = property on="Test Ring" class="Ring (strict)"("Visible"=TRUE) -> ()  [unwired: 2 in, 2 out]
                n199 = property on="Test Slider" class="Slide (strict)"("Visible"=FALSE) -> ()  [unwired: 2 in, 2 out]
              }
              frame "Exposure  **" {
                n200 = Index Array(array=w348, index=2) -> (element=w349:cluster{string[]})
                n201 = call <vilib>:"NT Read String.vi"("Name"=w351) -> ("String"=w350:string)  [unwired: 9 in, 1 out]
                n202 = Unbundle(w349) -> (w345:string[])
                n203 = Match First String(2:w345, 3:w350) -> (0:w346:i32)  [unwired: 1 out]
                n204 = property on="Test Ring" class="Ring (strict)"("Value"=w346, "Strings []"=w345) -> ()  [unwired: 2 in, 2 out]
                n205 = property on="Test Ring" class="Ring (strict)"("Visible"=TRUE) -> ()  [unwired: 2 in, 2 out]
                n206 = property on="Test Slider" class="Slide (strict)"("Visible"=FALSE) -> ()  [unwired: 2 in, 2 out]
              }
              frame "Exposure Priority  **" {
                n207 = Index Array(array=w357, index=3) -> (element=w358:cluster{string[]})
                n208 = call <vilib>:"NT Read String.vi"("Name"=w360) -> ("String"=w359:string)  [unwired: 9 in, 1 out]
                n209 = Unbundle(w358) -> (w354:string[])
                n210 = Match First String(2:w354, 3:w359) -> (0:w355:i32)  [unwired: 1 out]
                n211 = property on="Test Ring" class="Ring (strict)"("Value"=w355, "Strings []"=w354) -> ()  [unwired: 2 in, 2 out]
                n212 = property on="Test Ring" class="Ring (strict)"("Visible"=TRUE) -> ()  [unwired: 2 in, 2 out]
                n213 = property on="Test Slider" class="Slide (strict)"("Visible"=FALSE) -> ()  [unwired: 2 in, 2 out]
              }
              frame "Color Enable  **" {
                n214 = Index Array(array=w366, index=4) -> (element=w367:cluster{string[]})
                n215 = call <vilib>:"NT Read String.vi"("Name"=w369) -> ("String"=w368:string)  [unwired: 9 in, 1 out]
                n216 = Unbundle(w367) -> (w363:string[])
                n217 = Match First String(2:w363, 3:w368) -> (0:w364:i32)  [unwired: 1 out]
                n218 = property on="Test Ring" class="Ring (strict)"("Value"=w364, "Strings []"=w363) -> ()  [unwired: 2 in, 2 out]
                n219 = property on="Test Ring" class="Ring (strict)"("Visible"=TRUE) -> ()  [unwired: 2 in, 2 out]
                n220 = property on="Test Slider" class="Slide (strict)"("Visible"=FALSE) -> ()  [unwired: 2 in, 2 out]
              }
              frame Default {
                n221 = property on="Test Ring" class="Ring (strict)"("Visible"=FALSE) -> ()  [unwired: 2 in, 2 out]
                n222 = property on="Test Slider" class="Slide (strict)"("Visible"=FALSE) -> ()  [unwired: 2 in, 2 out]
              }
              frame "Brightness  **", "Color Level  **", "Compression  **", "FPS  **", "Sharpness  **" {
                n223 = call <vilib>:"NT Read Number.vi"("Name"=w375) -> ("Numeric"=w374:dbl)  [unwired: 9 in, 1 out]
                n224 = local write "Test Slider"(w374) -> ()
                n225 = property on="Test Slider" class="Slide (strict)"("Visible"=TRUE, "Scale.Maximum"=100.0 ("Scale.Range:Maximum")) -> ()  [unwired: 2 in, 2 out]
                n226 = property on="Test Ring" class="Ring (strict)"("Visible"=FALSE) -> ()  [unwired: 2 in, 2 out]
              }
            }
          }
        }
        n227 = property on="Progress" class="Clust (strict)"("Visible"=FALSE) -> ()  [unwired: 2 in, 2 out]
      }
      event "Test Name": Mouse Enter {
        # "Populate the ring with the list of tests"
        n228 = event-data() -> ()  [unwired: 1 in, 1 out]
        n229 = call <vilib>:"NT Read String Array.vi"("Name"="TestMode/TestList") -> ("String Array"=w383:string[])  [unwired: 9 in, 1 out]
        n230 = Build Array (concatenate)("Select the test to run...", w383) -> (w382:string[])
        n231 = property on="Test Name" class="Ring (strict)"("Strings []"=w382) -> ()  [unwired: 2 in, 2 out]
      }
      event "Test Name": Value Change {
        w385 = FALSE ("Visible")
        # "Tell the robot the test name to run"
        n232 = event-data() -> ("NewVal"=w389:u16)  [unwired: 1 in]
        n233 = property on="Test Name" class="Ring (strict)"() -> ("Strings []"=w390:string[])  [unwired: 2 in, 2 out]
        n234 = local write "Progress"(T7 {"Test Progress"=0, "Test Progress Text"=""} ("Progress")) -> ()
        n235 = Index Array(array=w390, index=w389) -> (element=w388:string)
        n236 = call <vilib>:"NT Write String.vi"("String"=w388, "Name"="TestMode/TestName") -> ()  [unwired: 9 in, 1 out]
        n237 = property on="Progress" class="Clust (strict)"("Visible"=TRUE) -> ()  [unwired: 2 in, 2 out]
        n238 = property on="Motor" class="Clust (strict)"("Visible"=w385) -> ()  [unwired: 2 in, 2 out]
        n239 = property on="Test Slider" class="Slide (strict)"("Visible"=w385) -> ()  [unwired: 2 in, 2 out]
        n240 = property on="On/Off" class="Bool (strict)"("Visible"=w385) -> ()  [unwired: 2 in, 2 out]
        n241 = property on="Rev/Fwd" class="Clust (strict)"("Visible"=w385) -> ()  [unwired: 2 in, 2 out]
        n242 = property on="Test Ring" class="Ring (strict)"("Visible"=w385) -> ()  [unwired: 2 in, 2 out]
      }
      event Mouse Enter {
        # "Populate the combo box with the list of autonomous options"
        n243 = event-data() -> ()  [unwired: 1 in, 1 out]
        n244 = call <vilib>:"NT Read String Array.vi"("Name"="Auto List") -> ("String Array"=w392:string[])  [unwired: 9 in, 1 out]
        n245 = property on="Select Auto" class="CmbBox (strict)"("Strings[]"=w392) -> ()  [unwired: 2 in, 2 out]
      }
      event Value Change {
        # "User modified the Auto Selection. Write to NT variable so robot knows."
        n246 = event-data() -> ("NewVal"=w395:T3)  [unwired: 1 in]
        n247 = call <vilib>:"NT Write String.vi"("String"=w395, "Name"="Auto Selector") -> ()  [unwired: 9 in, 1 out]
      }
      event "Command Selection": Value Change {
        # "Get the params and show in table"
        n248 = event-data() -> ("NewVal"=w401:i32)  [unwired: 1 in]
        n249 = property on="Command Selection" class="MCListbox (strict)"() -> ("ItemNames"=w399:string[][])  [unwired: 2 in, 2 out]
        n250 = call <vilib>:"WPI_DashboardUpdate Command Params.vi"("NewVal"=w401, "Commands"=w399, "Param Tbl"=w400) -> ()  [unwired: 8 in, 1 out]
      }
      event "Execute Command": Value Change {
        # "Started one, Unique ID holds\nresponse"
        n251 = event-data() -> ()  [unwired: 1 in, 1 out]
        n252 = property on="Command Selection" class="MCListbox (strict)"() -> ("ItemNames"=w412:string[][])  [unwired: 2 in, 2 out]
        n253 = Index Array(array=w412, index (row)="Command Selection", index (col)=0) -> (element=w410:string)
        n254 = call <vilib>:"Invoke Commands.vi"("Command Params"="Command Params", "Function Name"=w410) -> ("Params"=w406:u8, "Started"=w405:bool)  [unwired: 7 in, 1 out]
        n255 = Array Subset(array="Command Params", length (row)=w406) -> (w407:string[][])  [unwired: 3 in]
        n256 = Select(t="Executing" ("Cmd Status"), s=w405, f="" ("Cmd Status")) -> (s? t:f=→"Cmd Status":string)
      }
      event "Command Selection": Double Click {
        n257 = event-data() -> ("Row"=w420:i32)  [unwired: 1 in]
        n258 = property on="Command Selection" class="MCListbox (strict)"() -> ("ItemNames"=w423:string[][])  [unwired: 2 in, 2 out]
        n259 = local read "Command Params"() -> (w419:string[][])
        n260 = Index Array(array=w423, index (row)=w420, index (col)=0) -> (element=w421:string)
        n261 = call <vilib>:"Invoke Commands.vi"("Command Params"=w419, "Function Name"=w421) -> ("Params"=w418:u8, "Started"=w413:bool)  [unwired: 7 in, 1 out]
        n262 = Array Subset(array=w419, length (row)=w418) -> (w417:string[][])  [unwired: 3 in]
        n263 = Select(t="Executing" ("Cmd Status"), s=w413, f="" ("Cmd Status")) -> (s? t:f=w414:string)
        n264 = local write "Cmd Status"(w414) -> ()
      }
      event "CheckList": Double Click {
        # "Shift clears all"
        # "Update symbols on the listbox"
        n265 = event-data() -> ("PlatMods.Shift"=w425:bool, "Row"=w427:i32)  [unwired: 1 in]
        n266 = case shown="True" w425 {
          tunnel: w427 -> [w431 _]
          tunnel: 1 -> [w430 _]
          frame False {
            n267 = property on="CheckList" class="LstBox (strict)"() -> ("Item Symbols"=w429:i32[])  [unwired: 2 in, 2 out]
            n268 = Replace Array Subset(array=w429, new element=w430, index=w431) -> (w428:i32[])
            n269 = property on="CheckList" class="LstBox (strict)"("Item Symbols"=w428) -> ()  [unwired: 2 in, 2 out]
          }
          frame True {
            w432 = 0 ("Top Row")
            n270 = property on="CheckList" class="LstBox (strict)"() -> ("Number of Rows"=w434:u32)  [unwired: 2 in, 2 out]
            n271 = Initialize Array(0, w434) -> (w433:i32[])
            n272 = property on="CheckList" class="LstBox (strict)"("Top Row"=w432, "Value"=w432, "Item Symbols"=w433) -> ()  [unwired: 2 in, 2 out]
          }
        }
      }
      event "CheckList": Key Down {
        # "Update symbols on the listbox\nLeft and right keys check and uncheck"
        n273 = event-data() -> ("VKey"=w438:T23)  [unwired: 1 in]
        n274 = case shown="\"Left\", \"Right\"" w438 {
          selector: w438 -> [w443 _]
          tunnel: eventvkey."Left" ("VKey") -> [w441 _]
          frame "Left", "Right" {
            n275 = Equal?(x=w441, y=w443) -> (x = y?=w442:bool)
            n276 = Select(t=0, s=w442, f=1) -> (s? t:f=w444:i32)
            n277 = property on="CheckList" class="LstBox (strict)"() -> ("Item Symbols"=w447:i32[])  [unwired: 2 in, 2 out]
            n278 = Replace Array Subset(array=w447, new element=w444, index="CheckList") -> (w446:i32[])
            n279 = property on="CheckList" class="LstBox (strict)"("Item Symbols"=w446) -> ()  [unwired: 2 in, 2 out]
          }
          frame Default {
          }
        }
      }
      event "Motor.Enable": Value Change {
        # "When the test mode otor enable helper is set, update that\ntree row item's value"
        n280 = event-data() -> ("NewVal"=w453:bool)  [unwired: 1 in]
        n281 = Unbundle("Motor") -> ("Value"=w452:dbl)  [unwired: 1 out]
        n282 = Select(t=w452, s=w453, f=0.0) -> (s? t:f=w450:dbl)
        n283 = call <vilib>:"NT Write Number.vi"("Numeric"=w450, "Name"=w449) -> ()  [unwired: 9 in, 1 out]
      }
      event "Test Slider": Value Change {
        # "When the test mode slider helper is set, update that\ntree row item's value"
        n284 = event-data() -> ("NewVal"=w456:dbl)  [unwired: 1 in]
        n285 = call <vilib>:"NT Write Number.vi"("Numeric"=w456, "Name"=w457) -> ()  [unwired: 9 in, 1 out]
      }
      event "On/Off": Value Change {
        # "When the test mode on/off helper value is set, update that\ntree row item's value"
        n286 = event-data() -> ("NewVal"=w461:bool)  [unwired: 1 in]
        n287 = Boolean To (0,1)(Boolean=w461) -> (0, 1=w460:i16)
        n288 = call <vilib>:"NT Write Number.vi"("Numeric"=w460, "Name"=w459) -> ()  [unwired: 9 in, 1 out]
      }
      event "Rev/Fwd": Value Change {
        # "When the test mode helper value for relays is set, update that\ntree row item's value"
        n289 = event-data() -> ("NewVal.Forward"=w469:bool, "NewVal.Reverse"=w468:bool)  [unwired: 1 in]
        n290 = Boolean To (0,1)(Boolean=w469) -> (0, 1=w465:i16)
        n291 = Boolean To (0,1)(Boolean=w468) -> (0, 1=w467:i16)
        n292 = Negate(x=w467) -> (-x=w466:i16)
        n293 = Add(x=w465, y=w466) -> (x+y=w464:i16)
        n294 = call <vilib>:"NT Write Number.vi"("Numeric"=w464, "Name"=w463) -> ()  [unwired: 9 in, 1 out]
      }
      event "Test Ring": Value Change {
        # "When a test mode helper value is selected from the ring,\nset the tree item's variable to the string value"
        n295 = event-data() -> ("NewVal"=w473:u16)  [unwired: 1 in]
        n296 = property on="Test Ring" class="Ring (strict)"() -> ("Strings []"=w474:string[])  [unwired: 2 in, 2 out]
        n297 = Index Array(array=w474, index=w473) -> (element=w472:string)
        n298 = call <vilib>:"NT Write String.vi"("String"=w472, "Name"=w471) -> ()  [unwired: 9 in, 1 out]
      }
      event "Rec Mode": Value Change {
        # "Update globals for recording mode and path to read log from.\nClear when logging and let NetworkTables set path for vision to\nuse."
        n299 = event-data() -> ("NewVal"=w485:enum32{"Stop", "Record", "Playback"})  [unwired: 1 in]
        n300 = global write "WPI_DashboardLogging Global.vi" "Logging Filename"(path "") -> ()
        n301 = global write "WPI_DashboardLogging Global.vi" "Recording"(w485) -> ()
        n302 = case shown="\"Playback\"" w485 {
          tunnel: w484 -> [_ w487 w496]
          tunnel: [_ _ w495] -> w482
          tunnel: [_ _ w494] -> _
          tunnel: w480 -> [_ _ w492]
          tunnel: cluster{i32, i32} {-250, 170} -> [_ _ w491]
          tunnel: [_ _ T24 {"Image Size"=TRUE, "Image Type"=TRUE, "Pixel Value"=TRUE, "ROI Information"=TRUE, "Zoom Factor"=FALSE} ("Image Information Shown:All Elements")] -> w475
          tunnel: [_ _ TRUE ("Zoom Factor")] -> w476
          tunnel: w478 -> [_ _ w488]
          frame Default {
          }
          frame "Stop", "Record" {
            # "Place Window too"
            n303 = invoke class="VI" method="FP.Close"(reference=w487) -> (reference out=w486:refnum<vi>)  [unwired: 2 in, 2 out]
            n304 = invoke class="VI" method="Abort VI"(reference=w486) -> ()  [unwired: 2 in, 3 out]
          }
          frame "Playback" {
            n305 = call "Open Playback Panel.vi"("Offset"=w491, "DB VI Ref"=w492, "Playback in"=w496) -> ("Playback out"=w493:refnum<vi>)  [unwired: 8 in]
            n306 = register-events(w493, w488) -> (reference out=w495:refnum<event-registration>, error out=w494:errorcluster)  [unwired: 2 in]
          }
        }
        n307 = property on="Camera Image Right" class="ImageControl"("Image Information Shown"=w475, "Image Information Visible"=w476) -> ()  [unwired: 2 in, 2 out]
        n308 = property on="Camera Image" class="ImageControl"("Image Information Shown"=w475, "Image Information Visible"=w476) -> ()  [unwired: 2 in, 2 out]
        n309 = call <vilib>:"WPI_DashboardNT Log FieldName Cache.vi"("Operation"=enum16{"Lookup/Add", "Index", "Clear"}."Clear") -> ()  [unwired: 8 in, 3 out]
      }
      event Panel Close {
        w498 = enum32{"Stop", "Record", "Playback"}."Stop" ("Rec Mode")
        # "Playback window has been closed, abort"
        n310 = event-data() -> ()  [unwired: 1 in, 4 out]
        n311 = local write "Rec Mode"(w498) -> ()
        n312 = global write "WPI_DashboardLogging Global.vi" "Recording"(w498) -> ()
      }
      event Panel Close {
        # "Abort playback window and ourself"
        n313 = event-data() -> ()  [unwired: 1 in, 4 out]
        n314 = invoke class="VI" method="FP.Close"(reference=w502) -> (reference out=w501:refnum<vi>)  [unwired: 2 in, 2 out]
        n315 = invoke class="VI" method="Abort VI"(reference=w501) -> (error out=w500:errorcluster)  [unwired: 2 in, 2 out]
        n316 = invoke class="VI" method="Abort VI"(error in=w500) -> ()  [unwired: 2 in, 3 out]
      }
      event User Event {
        n317 = event-data() -> ("IDs"=w509:cluster{"RPC field ID":u16, "Unique ID":u16}, "String"=w508:string)  [unwired: 1 in]
        n318 = Bundle("IDs"=w509, "String"=w508) -> (w507:T10)  [unwired: 1 in]
        n319 = call <vilib>:"Retrieve RPC Response.vi"("RPC Response"=w507) -> ("Output"=w505:string[][])  [unwired: 10 in]
        n320 = Build Array (concatenate)(w503, w505) -> (w504:string[][])
        n321 = local write "Command Params"(w504) -> ()
        n322 = local write "Cmd Status"("" ("Cmd Status")) -> ()
      }
      event "Tree": Double Click {
        n323 = event-data() -> ("PlatMods"=w515:T27, "Tag"=w512:string)  [unwired: 1 in]
        n324 = Unbundle(w515) -> ("Shift"=w514:bool)  [unwired: 4 out]
        n325 = String Subset(string=w512, length (rest)=1 ("length (rest)")) -> (substring=w511:string)  [unwired: 1 in]
        n326 = Not(x=w514) -> (.not. x?=w513:bool)
        n327 = case shown="\"/\"" w511 {
          tunnel: w512 -> [_ w518]
          tunnel: w513 -> [_ w517]
          frame Default {
          }
          frame "/" {
            n328 = call <vilib>:"NT Update Persistence.vi"("Persistence"=w517, "Name"=w518) -> ()  [unwired: 9 in, 1 out]
          }
        }
      }
    }
  }
  n329 = while {
    tunnel: w68 -> [w520]
    i -> [w523]
    stop <- FALSE stop-if-true
    n330 = Wait (ms)(milliseconds to wait=u32 100) -> ()  [unwired: 1 out]
    n331 = case shown="\"Playback\"" "Rec Mode" {
      tunnel: w523 -> [_ _ w538]
      tunnel: [u32 2829099 ("Base Color") u32 11141120 ("Target Color") w527] -> w519
      frame "Stop", Default {
        # "Reset the color, extra updates don't cost much"
      }
      frame "Record" {
      }
      frame "Playback" {
        # "Playback"
        n332 = Quotient & Remainder(x=w538, y=u32 50 ("milliseconds to wait")) -> (x-y*floor(x/y)=w534:u32)  [unwired: 1 out]
        n333 = Divide(x=w534, y=u32 50 ("milliseconds to wait")) -> (x/y=w531:dbl)
        n334 = Multiply(x=6.283185307179586, y=w531) -> (x*y=w536:dbl)
        n335 = Sine(x=w536) -> (sin(x)=w535:dbl)
        n336 = Absolute Value(x=w535) -> (abs(x)=w528:dbl)
        n337 = call "Interpolate RGB Color.vi"("Proportion"=w528, "Target Color"=u32 30976, "Base Color"=u32 2829099) -> ("Result Color"=w527:u32)  [unwired: 8 in]
      }
    }
    n338 = property class="Pane"(reference=w520, "PaneColor"=w519) -> ()  [unwired: 1 in, 2 out]
  }
  n339 = call-poly <vilib>:"NT Read Value.vi"("Default Value"=FALSE, "Name"="Camera") -> ("Boolean"=w3:bool)  [unwired: 8 in, 1 out]
  n340 = case shown="True" w3 {
    tunnel: [T2."Drive" ("Dashboard Tab") T2."Camera" ("Dashboard Tab")] -> w35
    frame False {
    }
    frame True {
    }
  }
  n341 = local write "Dashboard Tab"(w35) -> ()
  n342 = property on="On/Off" class="Bool (strict)"("Visible"=w39) -> ()  [unwired: 2 in, 2 out]
  n343 = property on="Motor" class="Clust (strict)"("Visible"=w39) -> ()  [unwired: 2 in, 2 out]
  n344 = property on="Progress" class="Clust (strict)"("Visible"=w39) -> ()  [unwired: 2 in, 2 out]
  n345 = property on="Test Ring" class="Ring (strict)"("Visible"=w39) -> ()  [unwired: 2 in, 2 out]
  n346 = property on="Rev/Fwd" class="Clust (strict)"("Visible"=w39) -> ()  [unwired: 2 in, 2 out]
  n347 = local write "Command Selection"(u16 0 ("milliseconds to wait")) -> ()
  n348 = while {
    tunnel: u16 1741 ("timeout ms (25000)") -> [w542]
    stop <- FALSE stop-if-true
    n349 = TCP Create Listener(10:w542) -> (0:w541:errorcluster, 3:w543:refnum<k5>)  [unwired: 4 in, 1 out]
    n350 = case shown="No Error" w541 {
      selector: w541 -> [w545 _]
      tunnel: w543 -> [w546 _]
      frame No Error {
        n351 = while {
          tunnel: w546 -> [w549]
          tunnel: w545 -> [w548]
          stop <- FALSE stop-if-true
          n352 = TCP Wait On Listener(8:w548, 11:w549) -> (0:w550:errorcluster, 4:w551:refnum<k5>)  [unwired: 2 in, 3 out]
          n353 = local write "TCP"(w551) -> ()
          n354 = case shown="No Error" w550 {
            frame No Error {
            }
            frame Error {
              n355 = Wait (ms)(milliseconds to wait=u32 1000) -> ()  [unwired: 1 out]
            }
          }
        }
      }
      frame Error {
        n356 = Wait (ms)(milliseconds to wait=u32 1000) -> ()  [unwired: 1 out]
      }
    }
  }
  n357 = local write "Command Params"(string[][] [] ("Command Params")) -> ()
  n358 = global write "WPI_DashboardLogging Global.vi" "Recording"(w62) -> ()
  n359 = local write "Rec Mode"(w62) -> ()
  n360 = call <vilib>:"NT Write String.vi"("String"="Select Auto", "Name"="Auto Selector") -> ()  [unwired: 9 in, 1 out]
